vi "Numerical_Control_Prototype.vi"() -> ()   [LabVIEW 2017]
uses:
  <vilib>/OPCUA/controls/Write Status.ctl
  <vilib>/OPCUA/controls/NodeId.ctl
  <vilib>/OPCUA/client/Multiple Write Double.vi
  <vilib>/OPCUA/NI OPC UA Client.lvlib
panel:
  out "Temperature (C)":dbl
  in  "Temperature Control (C)":dbl(knob) scale=0.0..10.0
  out "Log Loop":i32
  out "Send Loop":i32
  in  "Stop Reading":bool
  in  "Node Status":T1 items=["Good"=0, "Uncertain_InitialValue"=1083310080, "Uncertain_LastUsableValue"=1083179008, "Uncertain_SensorNotAccurate"=1083375616, "Uncertain_EngineeringUnitsExceeded"=1083441152, "Bad_NoCommunication"=2150694912, "Bad_NotReadable"=2151284736, "Bad_NotWritable"=2151350272, "Bad_OutOfRange"=2151415808, "Bad_WaitingForInitialData"=2150760448]
  in  "Time Stamp":timestamp
  in  "Stop Control":bool
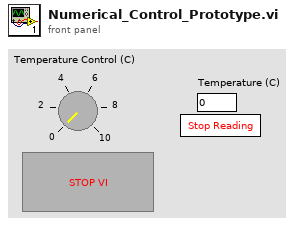
[diagram p1: front panel]
types:
  T1 = typedef "Write Status.ctl" = u32
  T2 = typedef "OPC UA Client Refnum.ctl" = refnum<k21>
  T3 = typedef "NodeId.ctl" = string
  T4 = cluster{"node ID":T3, "value":dbl, "timestamp (current time)":timestamp, "node status":T1}
  T5 = cluster{"node ID":T3, "value":dbl, "timestamp (current time)":timestamp, "node status":T1}[]
  T6 = typedef "Subscription ID.ctl" = u32
  T7 = typedef "Subscription Data Change.ctl" = cluster{"node ID":T3, " value":variant, "timestamp":timestamp, "data type":T8, "status code":T9}
  T8 = typedef "Data Type.ctl" = u16
  T9 = typedef "OPC UA StatusCode.ctl" = u32
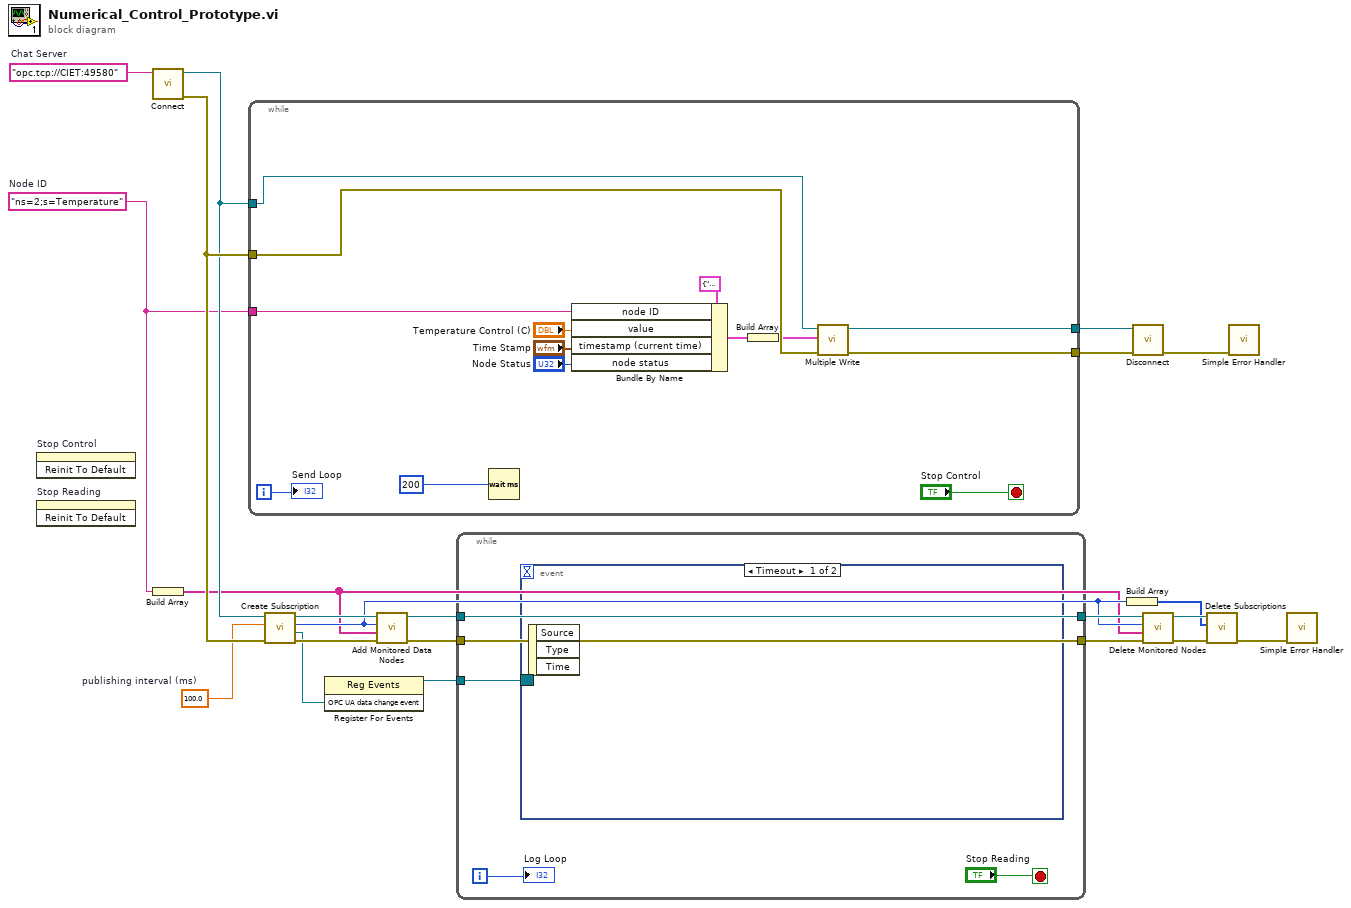
[diagram p0: block diagram]
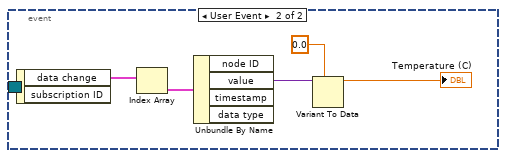
[diagram p2: hidden frame]
diagram:
  w1 = 100.0  # publishing interval (ms)
  w5 = "ns=2;s=Temperature"  # Node ID
  w21 = "opc.tcp://CIET:49580"  # Chat Server
  n1 = invoke on="Stop Control" class="Bool (strict)" method="Reinit To Default"() -> ()  [unwired: 3 in, 3 out]
  n2 = invoke on="Stop Reading" class="Bool (strict)" method="Reinit To Default"() -> ()  [unwired: 3 in, 3 out]
  n3 = call <vilib>:"Connect.vi"("server endpoint URL"=w21) -> ("error out"=w20:errorcluster, "OPC UA client refnum out"=w19:T2)  [unwired: 8 in, 1 out]
  n4 = Build Array(w5) -> (w4:string[])
  n5 = while {
    tunnel: w5 -> [w34]
    tunnel: w19 -> [w31]
    tunnel: w20 -> [w30]
    tunnel: [w33] -> w3
    tunnel: [w32] -> w2
    i -> [w35]
    stop <- "Stop Control" stop-if-true
    n6 = Wait (ms)(milliseconds to wait=u32 200) -> ()  [unwired: 1 out]
    n7 = Bundle By Name(cluster=T4 {"node ID"="", "value"=0.0, "timestamp (current time)"=timestamp(0 s since 1904-01-01), "node status"=0} ("request"), "node ID"=w34, "value"="Temperature Control (C)", "timestamp (current time)"="Time Stamp", "node status"="Node Status") -> (w25:T4)
    n8 = Build Array(w25) -> (w24:T5)
    n9 = call-poly <vilib>:"Multiple Write.vi"("error in (no error)"=w30, "requests"=w24, "OPC UA client refnum in"=w31) -> ("error out"=w32:errorcluster, "OPC UA client refnum out"=w33:T2)  [unwired: 5 in, 2 out]
    "Send Loop" <- w35
  }
  n10 = call <vilib>:"Create Subscription.vi"("error in (no error)"=w20, "publishing interval (1000 ms)"=w1, "OPC UA client refnum in"=w19) -> ("error out"=w17:errorcluster, "OPC UA data change event"=w16:refnum<user-event>, "subscription ID out"=w8:T6, "OPC UA client refnum out"=w18:T2)  [unwired: 4 in, 1 out]
  n11 = register-events(w16) -> (reference out=w15:refnum<event-registration>)  [unwired: 2 in, 1 out]
  n12 = call <vilib>:"Add Monitored Data Nodes.vi"("error in (no error)"=w17, "node IDs"=w4, "subscription ID in"=w8, "OPC UA client refnum in"=w18) -> ("error out"=w12:errorcluster, "OPC UA client refnum out"=w14:T2)  [unwired: 4 in, 2 out]
  n13 = while {
    tunnel: w15 -> [w41]
    tunnel: w14 -> [w39]
    tunnel: [w39] -> w13
    tunnel: w12 -> [w38]
    tunnel: [w38] -> w11
    i -> [w37]
    stop <- "Stop Reading" stop-if-true
    n14 = event shown="[0] Timeout" {
      selector: w41 -> [_ _]
      dyn-events: _ -> [_ _]
      timeout: _ -> [_ _]
      event Timeout {
        n15 = event-data() -> ()  [unwired: 1 in, 3 out]
      }
      event User Event {
        n16 = event-data() -> ("data change"=w46:T7[])  [unwired: 1 in, 1 out]
        n17 = Index Array(array=w46) -> (element=w45:T7)  [unwired: 1 in]
        n18 = Unbundle By Name(w45) -> ("value"=w44:variant)  [unwired: 3 out]
        n19 = Variant To Data(type=0.0, Variant=w44) -> (data=→"Temperature (C)":dbl)  [unwired: 1 in, 1 out]
      }
    }
    "Log Loop" <- w37
  }
  n20 = Build Array(w8) -> (w7:T6[])
  n21 = call <vilib>:"Disconnect.vi"("error in (no error)"=w2, "OPC UA client refnum in"=w3) -> ("error out"=w22:errorcluster)  [unwired: 9 in]
  n22 = call <vilib>:"Delete Monitored Nodes.vi"("error in (no error)"=w11, "node IDs"=w4, "subscription ID in"=w8, "OPC UA client refnum in"=w13) -> ("error out"=w9:errorcluster, "OPC UA client refnum out"=w10:T2)  [unwired: 3 in, 3 out]
  n23 = call <vilib>:"Delete Subscriptions.vi"("error in (no error)"=w9, "subscription IDs"=w7, "OPC UA client refnum in"=w10) -> ("error out"=w6:errorcluster)  [unwired: 6 in, 2 out]
  n24 = call <vilib>:"Simple Error Handler.vi"("error in (no error)"=w22) -> ()  [unwired: 4 in, 5 out]
  n25 = call <vilib>:"Simple Error Handler.vi"("error in (no error)"=w6) -> ()  [unwired: 4 in, 5 out]
